vi "Shutdown.vi"(8 "error in (no error)":errorcluster, 11 "Main in":refnum<class "Main.lvclass">) -> (0 "error out":errorcluster, 3 "Main out":refnum<class "Main.lvclass">)   [LabVIEW 2019, in "Main.lvclass"]
doc: "Developed by Kevin Thompson\nkevin@thompsonengineering.net\n\nCopyright 2018\nThompson Engineering, LLC"
uses:
  Main.lvclass
  Main.lvclass/Main.ctl
  Config/Config.lvclass/Config.ctl
  Accessors/Get Settings.vi
  Config/Accessors/Set Main Settings.vi
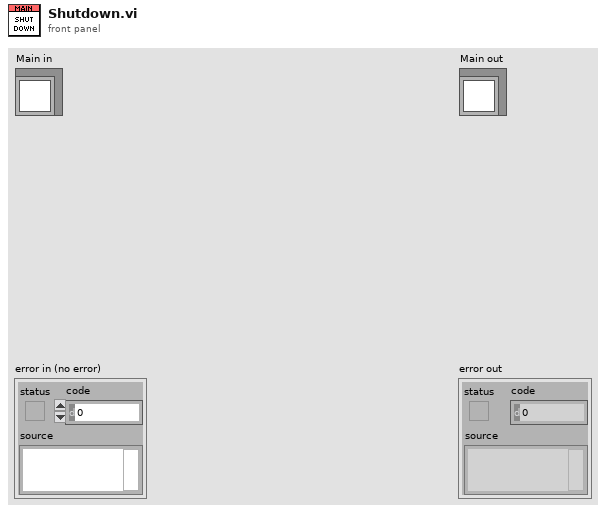
[diagram p1: front panel]
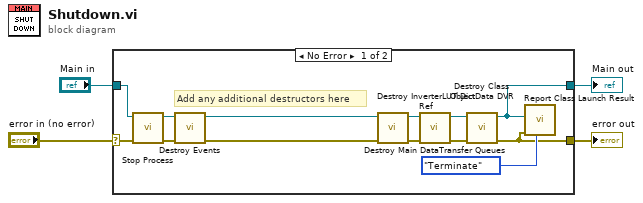
[diagram p0: block diagram]
diagram:
  n1 = case shown="No Error" "error in (no error)" {
    selector: "error in (no error)" -> [w5 w19]
    tunnel: [w13 w19] -> w3
    tunnel: [w14 w18] -> w1
    tunnel: "Main in" -> [w6 w18]
    frame No Error {
      # "Add any additional destructors here"
      n2 = call "Stop Process.vi"("error in (no error)"=w5, "Main in"=w6) -> ("error out"=w17:errorcluster, "Main out"=w16:refnum<class "Main.lvclass">)  [unwired: 8 in]
      n3 = call "Destroy Events.vi"("error in (no error)"=w17, "Main in"=w16) -> ("error out"=w10:errorcluster, "Main out"=w8:refnum<class "Main.lvclass">)  [unwired: 8 in]
      n4 = call "Destroy InverterLUT Dict Ref.vi"("error in (no error)"=w10, "Main in"=w8) -> ("error out"=w9:errorcluster, "Main out"=w7:refnum<class "Main.lvclass">)  [unwired: 8 in]
      n5 = call "Destroy Main DataTransfer Queues.vi"("error in (no error)"=w9, "Main in"=w7) -> ("error out"=w12:errorcluster, "Main out"=w11:refnum<class "Main.lvclass">)  [unwired: 8 in]
      n6 = call "Destroy Class ObjectData DVR.vi"("error in (no error)"=w12, "Main in"=w11) -> ("error out"=w13:errorcluster, "Main out"=w14:refnum<class "Main.lvclass">)  [unwired: 8 in]
      n7 = call "Report Class Launch Result.vi"("Object"=w14, "error in (no error)"=w13, "Mode (Launch)"=enum16{"Launch", "Terminate"}."Terminate") -> ()  [unwired: 7 in, 1 out]
    }
    frame Error {
    }
  }
  "error out" <- w3
  "Main out" <- w1
